vi "manageQueues.vi"(8 "error in (no error)":errorcluster) -> (0 "error out":errorcluster)   [LabVIEW 2017, in "programControl.lvlib"]
uses:
  programControl.lvlib
  Queue/TypeDefs/message.ctl
  loggingModule/Queue/TypeDefs/message.ctl
  ErrorMonitor/Queue/TypeDefs/message.ctl
  loggingModule/loggingModule.lvlib
  ErrorMonitor/ErrorMonitor.lvlib
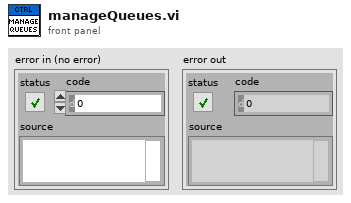
[diagram p1: front panel]
types:
  T1 = typedef "ErrorMonitor.lvlib/message.ctl" = cluster{"calling module":string, "message":string, "Data":variant}
  T2 = typedef "loggingModule.lvlib/message.ctl" = cluster{"calling module":string, "message":string, "data":variant}
  T3 = typedef "programControl.lvlib/message.ctl" = cluster{"calling module":string, "message":string, "Data":variant}
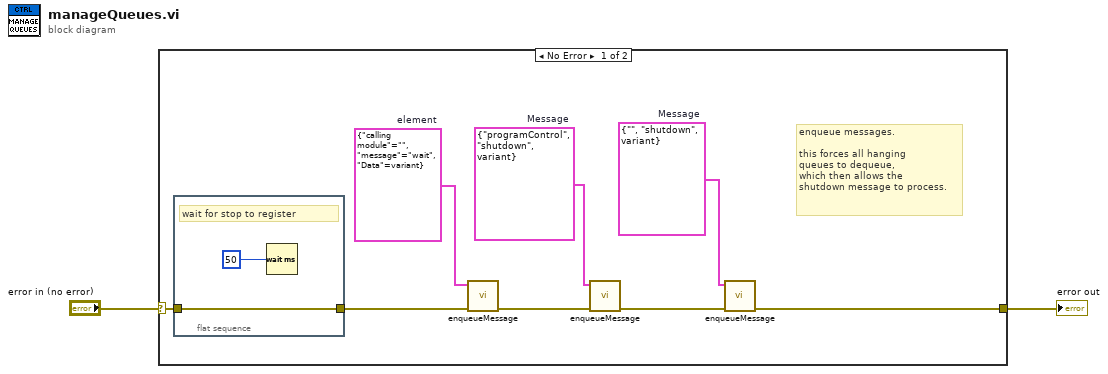
[diagram p0: block diagram]
diagram:
  n1 = case shown="No Error" "error in (no error)" {
    selector: "error in (no error)" -> [w10 w13]
    tunnel: [w6 w13] -> w1
    frame No Error {
      w3 = T1 {"calling module"="", "message"="shutdown", "Data"=variant}  # Message
      w4 = T2 {"calling module"="programControl", "message"="shutdown", "data"=variant}  # Message
      w5 = T3 {"calling module"="", "message"="wait", "Data"=variant}  # element
      # "enqueue messages.\n\nthis forces all hanging\nqueues to dequeue,\nwhich then allows the \nshutdown message to process."
      n2 = flat-sequence {
        tunnel: w10 -> [w12]
        tunnel: [w12] -> w9
        frame #0 {
          # "wait for stop to register"
          n3 = Wait (ms)(milliseconds to wait=u32 50) -> ()  [unwired: 1 out]
        }
      }
      n4 = call "enqueueMessage.vi"("error in (no error)"=w9, "element"=w5) -> ("error out"=w8:errorcluster)  [unwired: 9 in]
      n5 = call "enqueueMessage.vi"("error in (no error)"=w8, "Message"=w4) -> ("error out"=w7:errorcluster)  [unwired: 9 in]
      n6 = call "enqueueMessage.vi"("error in (no error)"=w7, "Message"=w3) -> ("error out"=w6:errorcluster)  [unwired: 9 in]
    }
    frame Error {
    }
  }
  "error out" <- w1
